vi "Counterweight.vi"() -> ()   [LabVIEW 2018]
uses:
  <vilib>/Analysis/polynomials.llb/Scalar Polynomial Evaluation (DBL).vi
  <vilib>/Analysis/NI_AALPro.lvlib
panel:
  in  "initialize":bool
  in  "Current Angle":dbl=-10.0 format="%#_13g"
  out "Current Counter Weight Power":dbl
  out "Counter Weight Power":dbl[](array[numeric])
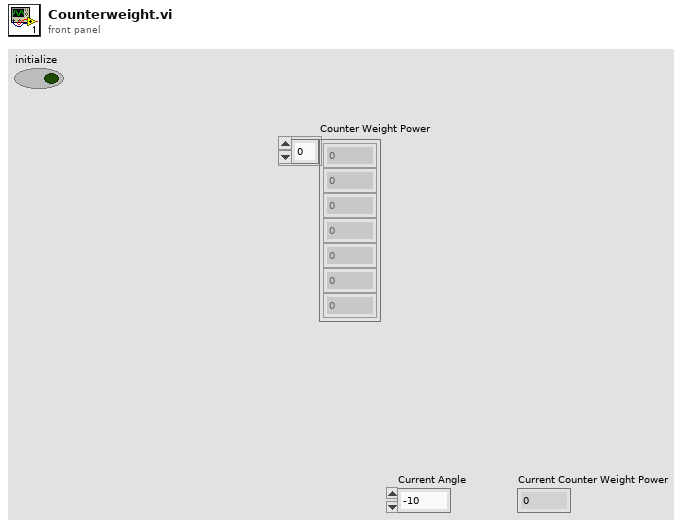
[diagram p1: front panel]
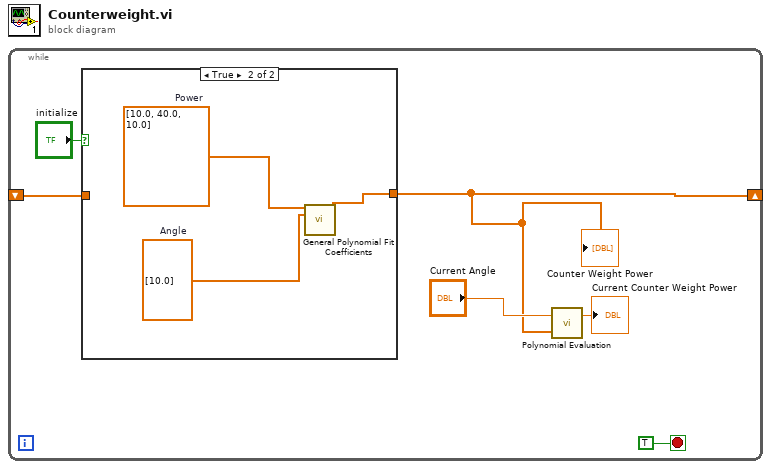
[diagram p0: block diagram]
diagram:
  n1 = while {
    shift-right: [w2] -> _
    shift-left: _ -> [w3]
    stop <- TRUE stop-if-true
    n2 = case shown="True" "initialize" {
      tunnel: [w7 w9] -> w2
      tunnel: w3 -> [w7 _]
      frame False {
      }
      frame True {
        w8 = dbl[] [10.0]  # Angle
        w10 = dbl[] [10.0, 40.0, 10.0]  # Power
        n3 = call <vilib>:"General Polynomial Fit Coefficients.vi"("Y"=w10, "X"=w8) -> ("Polynomial Coefficients"=w9:dbl[])  [unwired: 12 in, 1 out]
      }
    }
    "Counter Weight Power" <- w2
    n4 = call-poly <vilib>:"Polynomial Evaluation.vi"("P(x)"=w2, "a"="Current Angle") -> ("P(a)"=→"Current Counter Weight Power":dbl)  [unwired: 1 out]
  }
